vi "HistogramAnalysis.vi"(1 "coincidence settings":T3 {"center peak (µs)" format="%.2f"; "length [µs]" format="%.2f"}, 2 "ratio":bool, 3 "Array 2":T2(array[cluster]) {"offset (ns)" format="%.2f"; "origin (ns)" format="%.2f"}, 4 "threshold":u32) -> (0 "Array":dbl[][](array[numeric]) format="%.2f")   [LabVIEW 2009]
panel:
  out "Waveform Graph":T1(graph)
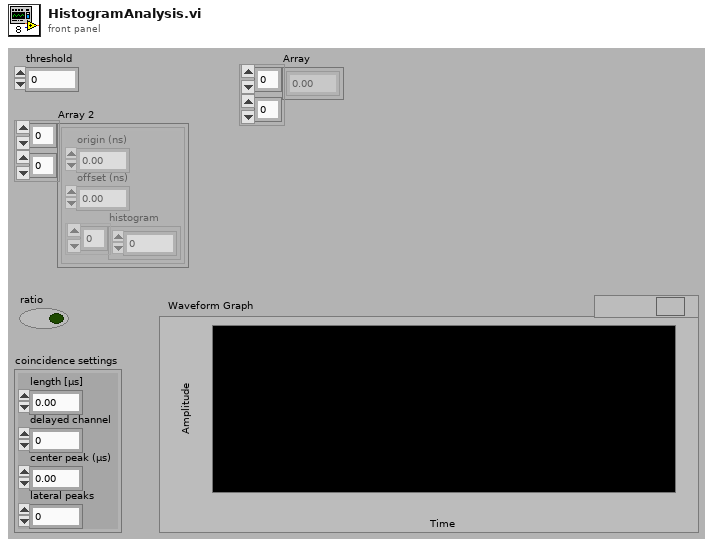
[diagram p1: front panel]
types:
  T1 = cluster{"origin (ns)":dbl, "offset (ns)":dbl, "histogram":u32[]}
  T2 = cluster{"origin (ns)":dbl, "offset (ns)":dbl, "histogram":u32[]}[][]
  T3 = cluster{"length [µs]":dbl, "delayed channel":u8, "center peak (µs)":dbl, "lateral peaks":u32}
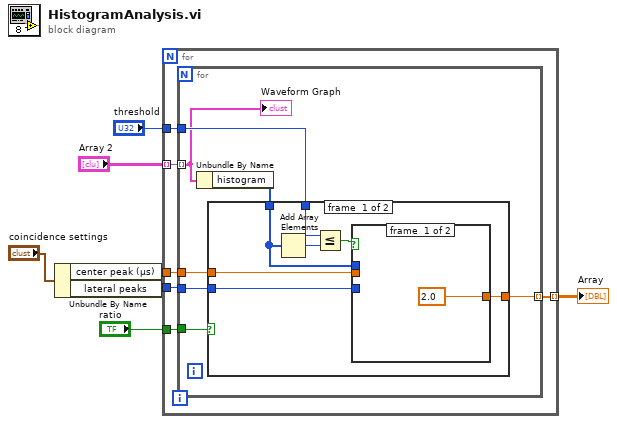
[diagram p0: block diagram]
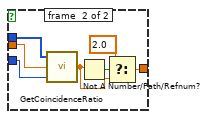
[diagram p2: hidden frame]
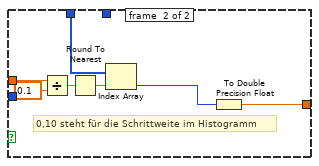
[diagram p3: hidden frame]
diagram:
  n1 = Unbundle By Name("coincidence settings") -> ("center peak (µs)"=w1:dbl, "lateral peaks"=w2:u32)
  n2 = for {
    tunnel: "ratio" -> [w13]
    tunnel: "threshold" -> [w12]
    tunnel: [w11] -> w5 mode=indexing
    tunnel: "Array 2" -> [w10] mode=indexing
    tunnel: w2 -> [w9]
    tunnel: w1 -> [w8]
    n3 = for {
      tunnel: w10 -> [w14] mode=indexing
      tunnel: [w20] -> w11 mode=indexing
      tunnel: w12 -> [w16]
      tunnel: w9 -> [w19]
      tunnel: w13 -> [w17]
      tunnel: w8 -> [w18]
      n4 = Unbundle By Name(w14) -> ("histogram"=w15:u32[])
      n5 = case shown="True" w17 {
        tunnel: [w27 w36] -> w20
        tunnel: w19 -> [w26 _]
        tunnel: w18 -> [w25 w42]
        tunnel: w16 -> [w22 _]
        tunnel: w15 -> [w21 w38]
        frame #0 {
          n6 = Add Array Elements(numeric array=w21) -> (sum=w24:u32)
          n7 = Less Or Equal?(x=w22, y=w24) -> (x <= y?=w23:bool)
          n8 = case shown="True" w23 {
            tunnel: [2.0 w33] -> w27
            tunnel: w26 -> [_ w32]
            tunnel: w25 -> [_ w31]
            tunnel: w21 -> [_ w30]
            frame #0 {
            }
            frame #1 {
              n9 = call "GetCoincidenceRatio.vi"("lateral peaks"=w32, "center peak (µs)"=w31, "histogram"=w30) -> ("coincidence ratio"=w29:dbl)
              n10 = Not A Number/Path/Refnum?(number/path/refnum=w29) -> (NaN/Path/Refnum?=w35:bool)
              n11 = Select(t=2.0, s=w35, f=w29) -> (s? t:f=w33:dbl)
            }
          }
        }
        frame #1 {
          # "0,10 steht für die Schrittweite im Histogramm"
          n12 = Divide(x=w42, y=0.1) -> (x/y=w40:dbl)
          n13 = Round To Nearest(number=w40) -> (nearest integer value=w39:dbl)
          n14 = Index Array(array=w38, index=w39) -> (element=w37:u32)
          n15 = To Double Precision Float(number=w37) -> (double precision float=w36:dbl)
        }
      }
      "Waveform Graph" <- w14
    }
  }
  "Array" <- w5
